vi "selection sorting.vi"(11 "input":dbl[](array[numeric])) -> (3 "sorted":dbl[](array[numeric]))   [LabVIEW 2014]
panel:
  out "Max":u32
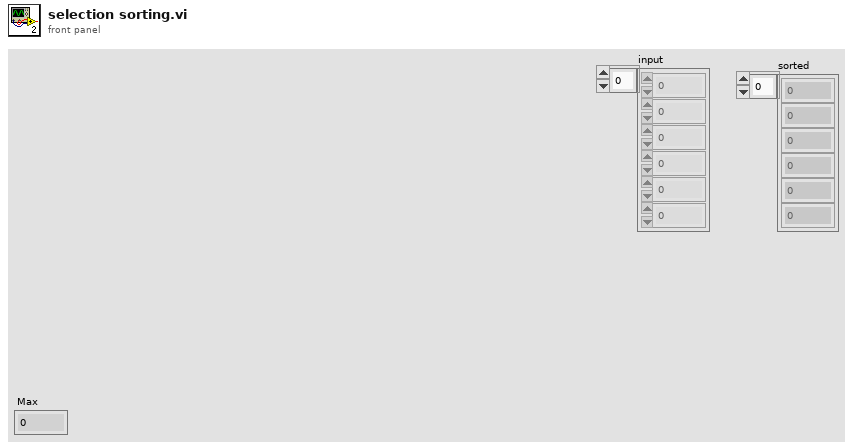
[diagram p1: front panel]
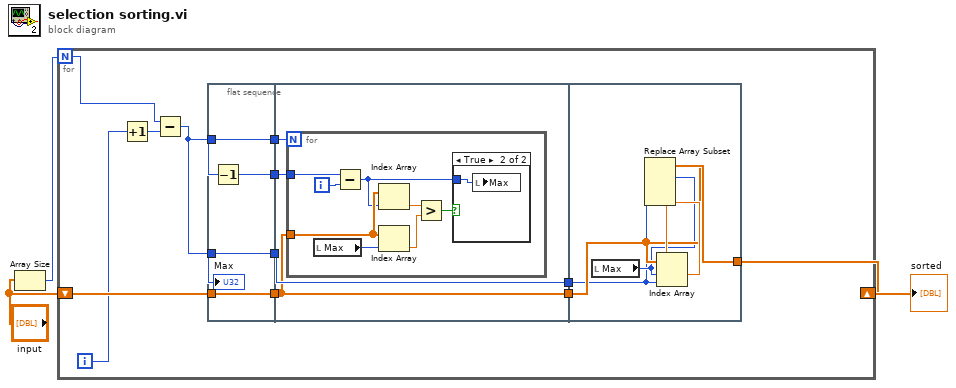
[diagram p0: block diagram]
diagram:
  n1 = Array Size(array="input") -> (size(s)=w3:i32)
  n2 = for {
    N: w3 -> [w6]
    shift-right: [w4] -> w2
    shift-left: "input" -> [w15]
    i -> [w8]
    n3 = Increment(x=w8) -> (x+1=w7:i32)
    n4 = Subtract(x=w6, y=w7) -> (x-y=w9:i32)
    n5 = flat-sequence {
      tunnel: w15 -> [w19]
      tunnel: [w19] -> w14
      tunnel: w9 -> [w16]
      tunnel: [w18] -> w11
      tunnel: w9 -> [w18]
      tunnel: [w17] -> w10
      tunnel: [w16] -> w5
      tunnel: w14 -> [w21]
      tunnel: [w21] -> w13
      tunnel: [w23] -> w12
      tunnel: w11 -> [w23]
      tunnel: w10 -> [w22]
      tunnel: w5 -> [w20]
      tunnel: w13 -> [w35]
      tunnel: w12 -> [w33]
      tunnel: [w36] -> w4
      frame #0 {
        n6 = Decrement(x=w16) -> (x-1=w17:i32)
        "Max" <- w18
      }
      frame #1 {
        n7 = for {
          N: w20 -> [_]
          tunnel: w21 -> [w30]
          tunnel: w22 -> [w26]
          i -> [w25]
          n8 = local read "Max"() -> (w31:u32)
          n9 = Subtract(x=w26, y=w25) -> (x-y=w24:i32)
          n10 = Index Array(array=w30, index=w24) -> (element=w28:dbl)
          n11 = Index Array(array=w30, index=w31) -> (element=w27:dbl)
          n12 = Greater?(x=w28, y=w27) -> (0:w29:bool)
          n13 = case shown="True" w29 {
            tunnel: w24 -> [_ w32]
            frame False {
            }
            frame True {
              n14 = local write "Max"(w32) -> ()
            }
          }
        }
      }
      frame #2 {
        n15 = local read "Max"() -> (w34:u32)
        n16 = Index Array(array=w35, index #1=w34, index #2=w33) -> (element #1=w37:dbl, element #2=w38:dbl)
        n17 = Replace Array Subset(array=w35, new element #1=w38, index #1=w34, new element #2=w37, index #2=w33) -> (w36:dbl[])
      }
    }
  }
  "sorted" <- w2
